vi "Set Unread Points in Buffer.vi"(9 "Set":bool, 10 "Value":u16) -> (2 "Value":u16)   [LabVIEW 2012]
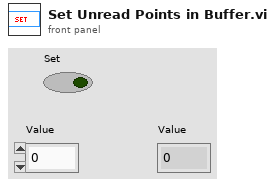
[diagram p1: front panel]
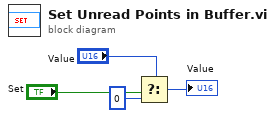
[diagram p0: block diagram]
diagram:
  n1 = Select(t="Value", s="Set", f=u16 0) -> (s? t:f=→"Value":u16)
